vi "Transmitter_RSMA - 3 SC - Timer & Modulation Config.vi"() -> ()   [LabVIEW 2022 SP3]
uses:
  <instrlib>/niUSRP/niUSRP Write Tx Data (CDB).vi
panel:
  out "SIG Size":i32
  in  "Iterations":i32=10000
  out "Time(s)":sgl format="%#_4g"
  in  "Beta/Alpha":dbl(slide)=0.04000000000000001 step=0.005 scale=0.0..1.0
  in  "Alpha":dbl(slide)=0.2 step=0.005 scale=0.0..1.0
  in  "Tab Control":enum32{"USRP Parameters", "Transmission"}(tab)
  in  "USRP ControledParameters 2":T1={"Active Antenna"="TX1", "Gain (dB)"=0.0, "Carrier Frequency"=2400000000.0, "IQ Rate"=2000000.0, "Active Channel"="0"} {"IQ Rate" format="%#_6p"; "Carrier Frequency" format="%#_6p"; "Gain (dB)" format="%#_6f"}
  in  "Device selection":refnum<k15>="RIO0"
  in  "stop":bool
  in  "Common Bits":i32=3
  in  "Total Bits":i32=6
  out "Error out":errorcluster
  in  "Modulation parameter":T2={"Modulation type"=enum."QPSK(4QAM)", "BCC rate (k/n)"=enum."1/2", "Modulation 2"=enum."BPSK", "Modulation 3"=enum."BPSK"}
  out "Bits length":i32
  out "Bits length 2":i32
  out "Frame Duration":dbl format="%#_6p"
  out "Coerced Parameters":T3={"IQ Rate"=100000.0, "Carrier  Freq."=100000.0, "Gain"=0.0} {"Gain" format="%#_6f"; "Carrier  Freq." format="%#_6p"; "IQ Rate" format="%#_6p"}
  out "Transmitted Waveform":dbl[](graph)
  in  "Message 2":string="ptua. At vero eos et accusam et justo duo dolores et ea rebum. Stet clita kasd gubergren, no sea takimata sanctus est Lorem ipsum dolor sit amet. Lore"
  in  "Message 1":string="Lorem ipsum dolor sit amet, consetetur sadipscing elitr, sed diam nonumy eirmod tempor invidunt ut labore et dolore magna aliquyam erat, sed diam volu"
  in  "error in (no error)":errorcluster
  # "RSMA Transmitter"
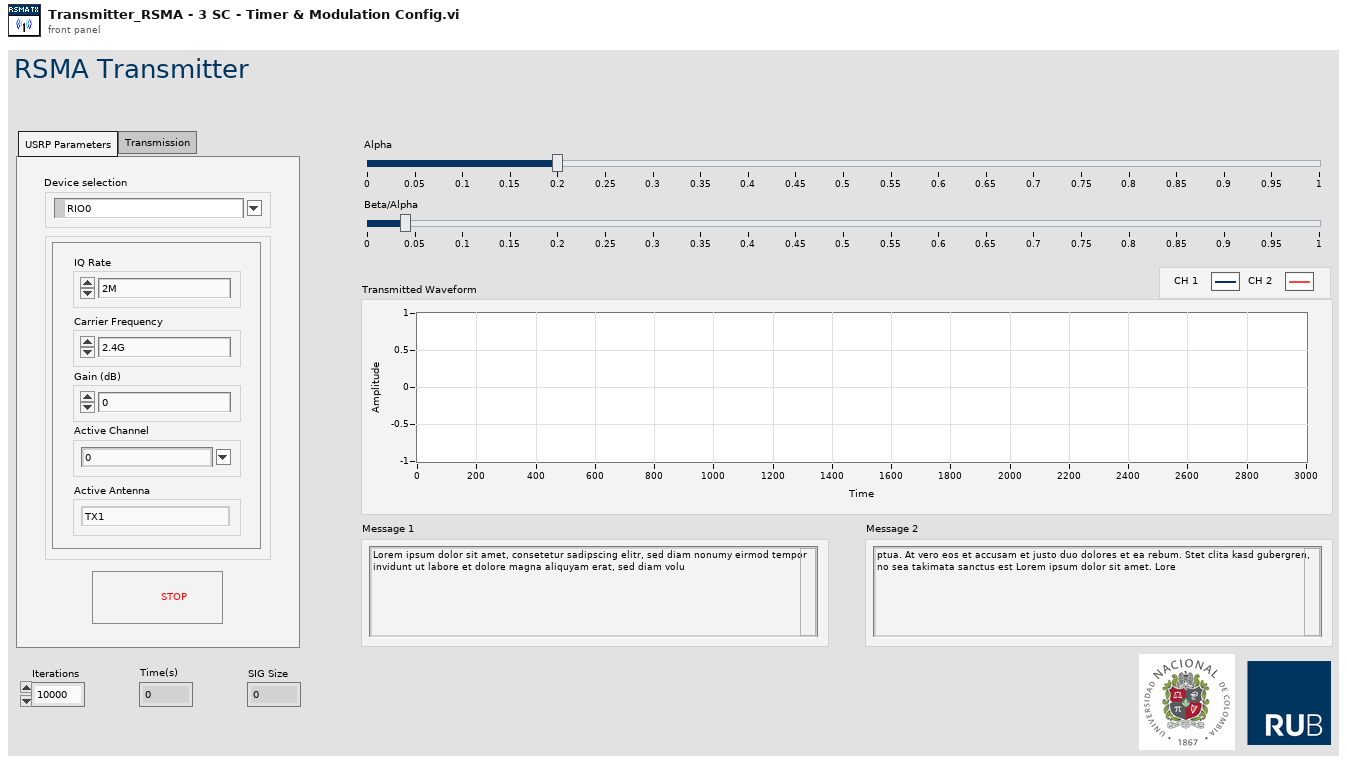
[diagram p1: front panel]
types:
  T1 = cluster{"Active Antenna":string, "Gain (dB)":dbl, "Carrier Frequency":dbl, "IQ Rate":dbl, "Active Channel":string}
  T2 = cluster{"Modulation type":enum16{"QPSK(4QAM)", "64QAM", "16QAM", "BPSK", "BPSK Vertical"}, "BCC rate (k/n)":enum16{"1/2", "2/3", "3/4"}, "Modulation 2":enum16{"QPSK(4QAM)", "64QAM", "16QAM", "BPSK", "BPSK Vertical"}, "Modulation 3":enum16{"QPSK(4QAM)", "64QAM", "16QAM", "BPSK", "BPSK Vertical"}}
  T3 = cluster{"IQ Rate":dbl, "Carrier  Freq.":dbl, "Gain":dbl}
  T4 = cluster{"coerced IQ rate":dbl, "coerced carrier frequency":dbl, "coerced gain":dbl}
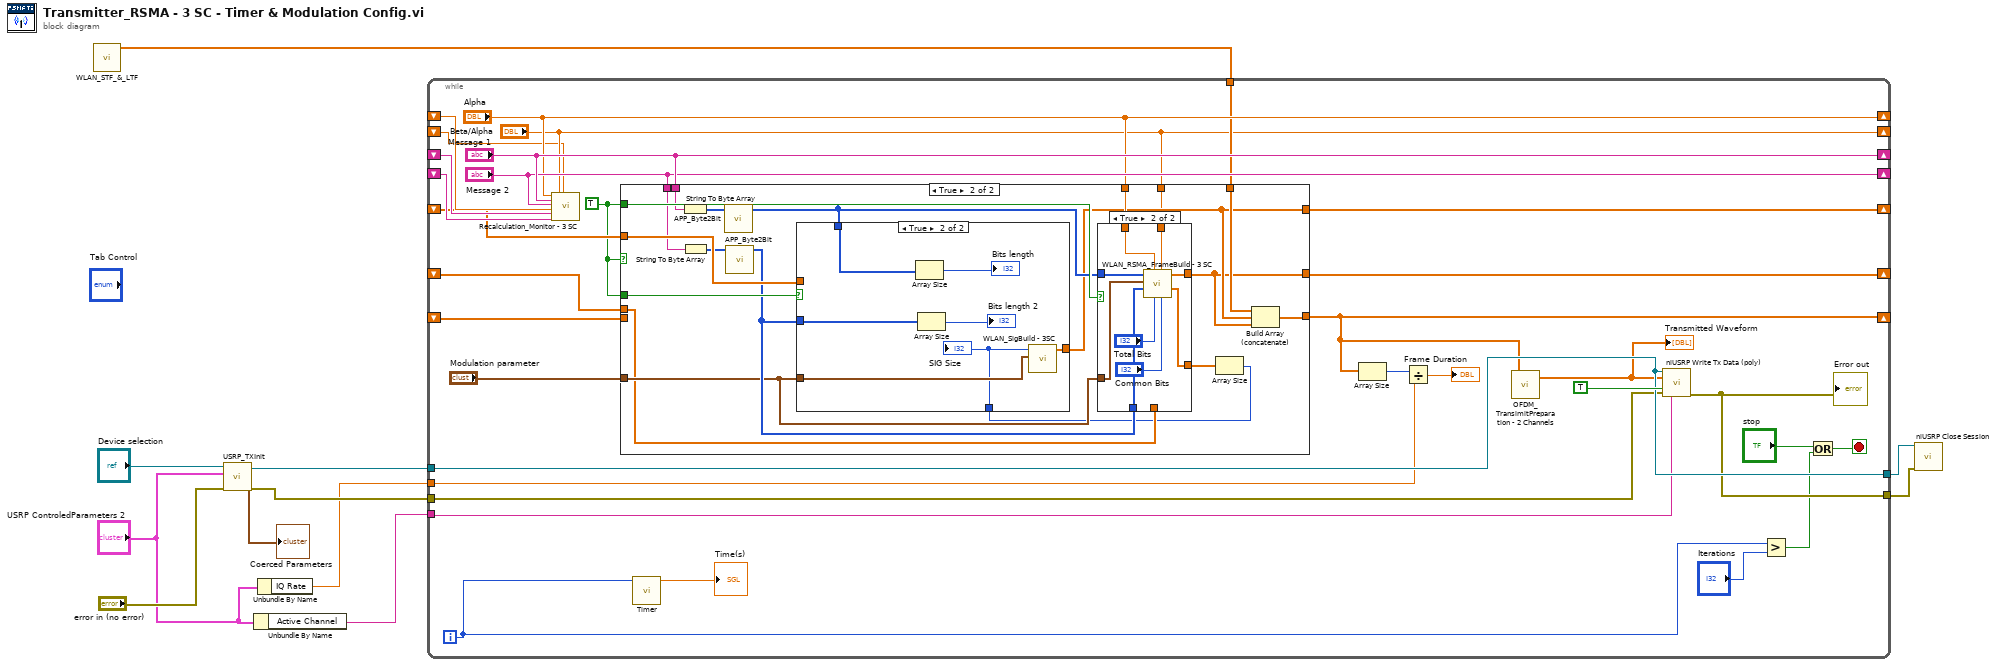
[diagram p0: block diagram]
diagram:
  n1 = call "WLAN_STF_&_LTF.vi"() -> ("STF & LTF"=w1:cdb[])  [unwired: 11 in]
  n2 = call "USRP_TXInit.vi"("device names"="Device selection", "USRP ControledParameters"="USRP ControledParameters 2", "error in (no error)"="error in (no error)") -> ("session handle out"=w10:refnum<k15>, "USRP CoercedParamters"=→"Coerced Parameters":T4, "error out"=w9:errorcluster)  [unwired: 5 in]
  n3 = Unbundle By Name("USRP ControledParameters 2") -> ("Active Channel"=w2:string)
  n4 = Unbundle By Name("USRP ControledParameters 2") -> ("IQ Rate"=w8:dbl)
  n5 = while {
    tunnel: w10 -> [w40]
    tunnel: w9 -> [w24]
    tunnel: w8 -> [w39]
    tunnel: [w40] -> w7
    tunnel: [w38] -> w6
    tunnel: w2 -> [w37]
    shift-right: ["Alpha"] -> _
    shift-left: _ -> [w36]
    shift-right: ["Message 1"] -> _
    shift-left: _ -> [w35]
    shift-right: ["Message 2"] -> _
    shift-left: _ -> [w34]
    shift-right: [w31] -> _
    shift-left: _ -> [w30]
    shift-right: [w28] -> _
    shift-left: _ -> [w27]
    tunnel: w1 -> [w26]
    shift-right: [w23] -> _
    shift-left: _ -> [w25]
    shift-right: ["Beta/Alpha"] -> _
    shift-left: _ -> [w20]
    i -> [w15]
    stop <- w17 stop-if-true
    w12 = TRUE
    n6 = call "Recalculation_Monitor - 3 SC.vi"("Alpha"="Alpha", "Message 1"="Message 1", "Message 2"="Message 2", "Alpha old"=w36, "Message 1 old"=w35, "Message 2 old"=w34, "Beta/Alpha"="Beta/Alpha", "Beta/Alpha old"=w20) -> ()  [unwired: 9 in, 3 out]
    n7 = case shown="True" w12 {
      tunnel: w12 -> [_ w65]
      tunnel: w12 -> [_ w64]
      tunnel: "Message 1" -> [_ w59]
      tunnel: "Message 2" -> [_ w60]
      tunnel: "Modulation parameter" -> [_ w56]
      tunnel: [w46 w52] -> w31
      tunnel: w30 -> [w46 w63]
      tunnel: "Alpha" -> [_ w55]
      tunnel: [w45 w51] -> w28
      tunnel: w27 -> [w45 w54]
      tunnel: w26 -> [_ w53]
      tunnel: [w44 w50] -> w23
      tunnel: w25 -> [w44 _]
      tunnel: "Beta/Alpha" -> [_ w49]
      frame False {
      }
      frame True {
        n8 = String To Byte Array(string=w59) -> (unsigned byte array=w61:u8[])
        n9 = String To Byte Array(string=w60) -> (unsigned byte array=w62:u8[])
        n10 = call "APP_Byte2Bit.vi"("input byte stream"=w61) -> ("output bit stream"=w57:i8[])  [unwired: 10 in]
        n11 = call "APP_Byte2Bit.vi"("input byte stream"=w62) -> ("output bit stream"=w58:i8[])  [unwired: 10 in]
        n12 = case shown="True" w64 {
          tunnel: w58 -> [_ w75]
          tunnel: w57 -> [_ w74]
          tunnel: w56 -> [_ w73]
          tunnel: w55 -> [_ w72]
          tunnel: [w66 w70] -> w51
          tunnel: w54 -> [w66 _]
          tunnel: w49 -> [_ w71]
          tunnel: [w66 w69] -> w48
          frame False {
          }
          frame True {
            n13 = call "WLAN_RSMA_FrameBuild - 3 SC.vi"("Common Bits"="Common Bits", "Beta/Alpha"=w71, "Total Bits"="Total Bits", "Alpha"=w72, "data in 2"=w75, "Modulation parameter"=w73, "data in"=w74) -> ("Constellation Map"=w69:cdb[], "output array"=w70:cdb[])  [unwired: 2 in, 1 out]
          }
        }
        n14 = Array Size(array=w48) -> (size(s)=w47:i32)
        n15 = case shown="True" w65 {
          tunnel: w56 -> [_ w78]
          tunnel: [w76 w81] -> w52
          tunnel: w63 -> [w76 _]
          tunnel: w58 -> [_ w80]
          tunnel: w57 -> [_ w79]
          tunnel: w47 -> [_ w77]
          frame False {
          }
          frame True {
            n16 = Array Size(array=w79) -> (size(s)=→"Bits length":i32)
            n17 = Array Size(array=w80) -> (size(s)=→"Bits length 2":i32)
            n18 = call "WLAN_SigBuild - 3SC.vi"("Data bit length"=w77, "Modulation parameter"=w78) -> ("symbols"=w81:cdb[])  [unwired: 7 in, 1 out]
            "SIG Size" <- w77
          }
        }
        n19 = Build Array (concatenate)(w53, w52, w51) -> (w50:cdb[])
      }
    }
    n20 = call "Timer.vi"("index"=w15) -> ("Time(s)"=→"Time(s)":sgl)  [unwired: 10 in]
    n21 = Array Size(array=w23) -> (size(s)=w42:i32)
    n22 = Divide(x=w42, y=w39) -> (x/y=→"Frame Duration":dbl)
    n23 = call "OFDM_TransimitPreparation - 2 Channels.vi"("array"=w23) -> ("output array"=w22:cdb[])  [unwired: 8 in, 2 out]
    "Transmitted Waveform" <- w22
    n24 = call-poly <instrlib>:"niUSRP Write Tx Data (poly).vi"("session handle"=w40, "channel list"=w37, "data"=w22, "end of data?"=TRUE, "error in (no error)"=w24) -> ("error out"=w38:errorcluster)  [unwired: 9 in, 1 out]
    "Error out" <- w38
    n25 = Greater?(x=w15, y="Iterations") -> (0:w16:bool)
    n26 = Or(x="stop", y=w16) -> (x .or. y?=w17:bool)
  }
  n27 = call <instrlib>:"niUSRP Close Session.vi"("session handle"=w7, "error in (no error)"=w6) -> ()  [unwired: 13 in, 1 out]
